vi "使用范例_单行数据存储B.vi"() -> ()   [LabVIEW 2020]
panel:
  in  "文件头（最后一个字符是换行）":string="Current Voltage\nI V\n"
  in  "存储路径":path=path "D:/"
  in  "其他说明信息":string="300K_1000Oe"
  in  "测试项目":string="IVcurve"
  in  "样品名称":string="deviceUnderTest"
  in  "是否添加时间？":bool=TRUE
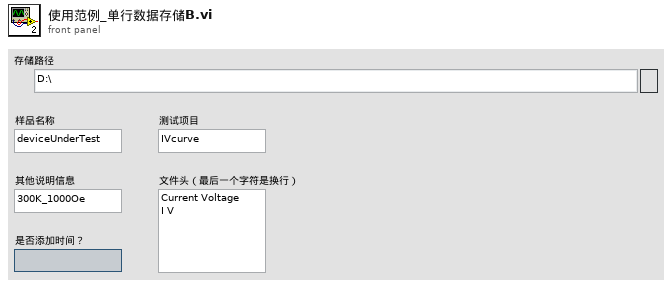
[diagram p1: front panel]
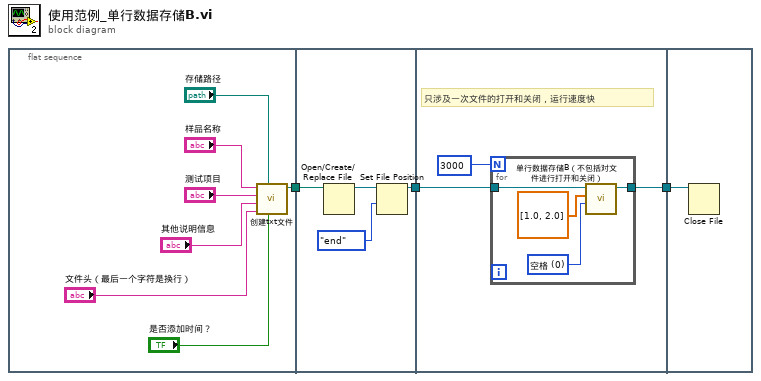
[diagram p0: block diagram]
diagram:
  n1 = flat-sequence {
    tunnel: [w4] -> w3
    tunnel: w3 -> [w12]
    tunnel: [w11] -> w2
    tunnel: w2 -> [w16]
    tunnel: [w15] -> w1
    tunnel: w1 -> [w22]
    frame #0 {
      n2 = call "创建txt文件.vi"("是否添加时间？"="是否添加时间？", "存储路径"="存储路径", "文件头（最后一个字符是换行）"="文件头（最后一个字符是换行）", "其他说明信息"="其他说明信息", "测试项目"="测试项目", "样品名称"="样品名称") -> ("文件路径"=w4:path)  [unwired: 5 in]
    }
    frame #1 {
      n3 = Open/Create/Replace File(file path (use dialog)=w12) -> (refnum out=w14:refnum<file>)  [unwired: 5 in, 2 out]
      n4 = Set File Position(refnum=w14, from (0:start)=enum16{"start", "end", "current"}."end" ("自（0:起始）")) -> (refnum out=w11:refnum<file>)  [unwired: 2 in, 1 out]
    }
    frame #2 {
      # "只涉及一次文件的打开和关闭，运行速度快"
      n5 = for {
        N: 3000 -> [_]
        tunnel: w16 -> [w21]
        tunnel: [w20] -> w15
        w19 = u16 0 items=["空格", "制表符"] ("分隔符")
        n6 = call "单行数据存储B（不包括对文件进行打开和关闭）.vi"("分隔符"=w19, "存储向量"=dbl[] [1.0, 2.0], "文件引用句柄输入"=w21) -> ("文件引用句柄输出"=w20:refnum<file>)  [unwired: 6 in]
      }
    }
    frame #3 {
      n7 = Close File(refnum=w22) -> ()  [unwired: 1 in, 2 out]
    }
  }
